vi "Pockels Cal-Reset cursors.vi"(8 "error in (no error)":errorcluster, 11 "XYGraph in":refnum<vi>) -> (0 "error out":errorcluster, 3 "XYGraph":refnum<vi>)   [LabVIEW 2020]
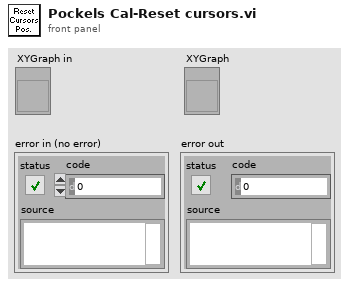
[diagram p1: front panel]
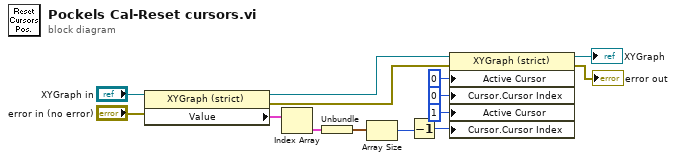
[diagram p0: block diagram]
diagram:
  n1 = property on="Property Node" class="XYGraph (strict)"(reference="XYGraph in", error in="error in (no error)") -> (reference out=w11:refnum<vi>, error out=w3:errorcluster, "Value"=w12:cluster{cluster{"Value":dbl, "Value":dbl}[]}[])
  n2 = Index Array(array=w12) -> (element=w13:cluster{cluster{"Value":dbl, "Value":dbl}[]})  [unwired: 1 in]
  n3 = Unbundle(w13) -> (w14:cluster{"Value":dbl, "Value":dbl}[])
  n4 = Array Size(array=w14) -> (size(s)=w9:i32)
  n5 = Decrement(x=w9) -> (x-1=w8:i32)
  n6 = property on="Property Node" class="XYGraph (strict)"(reference=w11, error in=w3, "Active Cursor"=u32 0, "Cursor.Cursor Index"=0, "Active Cursor"=u32 1, "Cursor.Cursor Index"=w8) -> (reference out=→"XYGraph":refnum<vi>, error out=→"error out":errorcluster)
